vi "dfd_Lattice AR Normalization (OneM).vi"(7 "scale type":T1, 10 "coefficients k":dbl[](array[numeric]) format="%.2f", 11 "x":dbl[](array[numeric])) -> (2 "norm":dbl[](array[numeric]) format="%.2f", 3 "y":dbl[](array[numeric]))   [LabVIEW 2017, in "NI_DigFilter_FXP.lvlib"]
uses:
  <vilib>/addons/Digital Filter Design/NI_DigFilter_FXP.lvlib
  <vilib>/addons/Digital Filter Design/_Objects.llb/DFD Coef Norm Type.ctl
  <vilib>/addons/Digital Filter Design/NI_DigFilterLicensed.lvlib
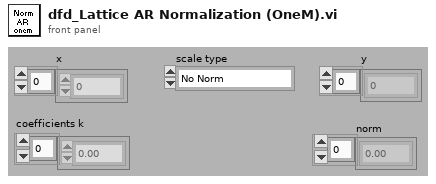
[diagram p1: front panel]
types:
  T1 = typedef "NI_DigFilterLicensed.lvlib/DFD Coef Norm Type.ctl" = enum16{"No Norm", "Time Domain 1-Norm", "Time Domain 2-Norm", "Time Domain Inf-Norm"}
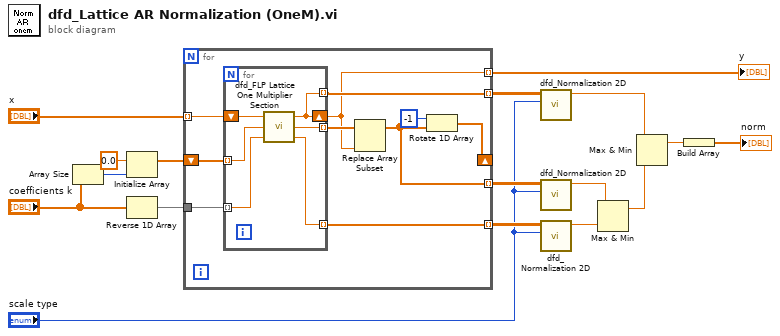
[diagram p0: block diagram]
diagram:
  n1 = Array Size(array="coefficients k") -> (size(s)=w15:i32)
  n2 = Initialize Array(0.0 ("element"), w15) -> (w17:dbl[])
  n3 = Reverse 1D Array(array="coefficients k") -> (reversed array=w14:dbl[])
  n4 = for {
    tunnel: w14 -> [w27]
    shift-right: [w26] -> _
    shift-left: w17 -> [w25]
    tunnel: [w19] -> w9 mode=indexing
    tunnel: [w24] -> w10 mode=indexing
    tunnel: [w23] -> w8 mode=indexing
    tunnel: "x" -> [w20] mode=indexing
    tunnel: [w18] -> w1 mode=indexing
    n5 = for {
      shift-right: [w29] -> w18
      shift-left: w20 -> [w33]
      tunnel: w25 -> [w32] mode=indexing
      tunnel: w27 -> [w31] mode=indexing
      tunnel: [w30] -> w22 mode=indexing
      tunnel: [w29] -> w24 mode=indexing
      tunnel: [w28] -> w23 mode=indexing
      n6 = call <vilib>:"dfd_FLP Lattice One Multiplier Section.vi"("k(m)"=w31, "w(m-1)"=w32, "x(m)"=w33) -> ("u(m)"=w28:dbl, "w(m)"=w30:dbl, "x(m-1)"=w29:dbl)
    }
    n7 = Replace Array Subset(array=w22, new element=w18) -> (w19:dbl[])  [unwired: 1 in]
    n8 = Rotate 1D Array(1:w19, 2:-1 ("n")) -> (0:w26:dbl[])
  }
  "y" <- w1
  n9 = call <vilib>:"dfd_Normalization 2D.vi"("scale type"="scale type", "2D Array (col-major)"=w10) -> ("max norm"=w4:dbl)  [unwired: 9 out]
  n10 = call <vilib>:"dfd_Normalization 2D.vi"("scale type"="scale type", "2D Array (col-major)"=w9) -> ("max norm"=w5:dbl)  [unwired: 9 out]
  n11 = call <vilib>:"dfd_Normalization 2D.vi"("scale type"="scale type", "2D Array (col-major)"=w8) -> ("max norm"=w6:dbl)  [unwired: 9 out]
  n12 = Max & Min(x=w5, y=w6) -> (max(x,y)=w3:dbl)  [unwired: 1 out]
  n13 = Max & Min(x=w4, y=w3) -> (max(x,y)=w2:dbl)  [unwired: 1 out]
  n14 = Build Array(w2) -> (→"norm":dbl[])
